vi "Dispense X Gallon at Y Flowrate.vi"(0 "Gallon Target":dbl=10.72, 1 "Equipment":T3={"COM Port"="COM1", "MW100"="MW100", "AG34970"="A-34972A", "Chamber"="WT500"}, 2 "Semiphore":T4, 5 "GPM Target":dbl=3.0, 11 "Error In":errorcluster, 12 "Test Condition":T1=enum."SRK500,Station1,5GPM FR", 13 "Ctl Refnum":refnum<vi>) -> (4 "M*-1":dbl, 6 "M*(Gallons)":dbl, 8 "ToutMax":dbl, 10 "ToutMin":dbl, 14 "POWER Ref":refnum<vi>, 15 "Error Out":errorcluster)   [LabVIEW 2009]
uses:
  PowerElements.ctl
  EquipReferences.ctl
  HEWH Tank Indicator.ctl
  TestedFlowratesScenarios.ctl
  Intellifaucet/Intellfaucet Mode.ctl
  ChannelSettings.ctl
panel:
  out "Tank Display":T2 {"TC6" format="%.2g"; "TIN" format="%.2g"; "TOUT" format="%.2g"; "Mean" format="%.2f"; "Std Dev" format="%.2f"; "TC5" format="%.2g"; "TC4" format="%.2g"; "TC3" format="%.2g"; "TC2" format="%.2g"; "TC1" format="%.2g"}
  out "String":string
  out "Flow":dbl=3.8899999999999997
  out "Flow Chart":dbl(graph)
  out "Local?":bool
  out "MW100":refnum<visa-resource-name>="MW100"
  out "POWER":T5
  out "Current Draw Start Time":dbl format="%.2f"
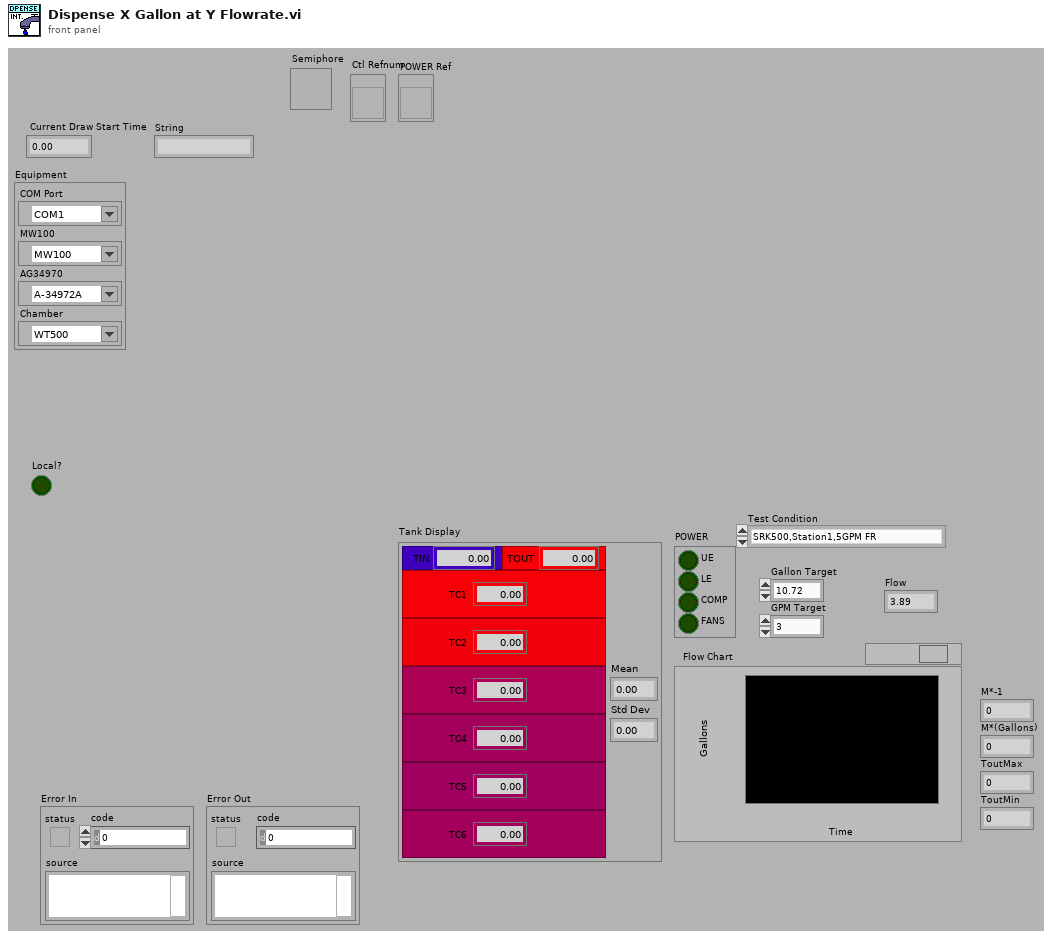
[diagram p1: front panel]
types:
  T1 = typedef "TestedFlowratesScenarios.ctl" = enum16{"DRK500,Station1", "DRK375,Lab", "SRK500,Station1,5GPM FR", "DRK375,STATION3,1/2\"HOSE", "DRK500,Station1,downspout", "DRK375,Station3,thruEcocute", "DRK375,Station3,purge", "Build2,2B,Purge", "Global, Purge", "Global, Tank"}
  T2 = typedef "HEWH Tank Indicator.ctl" = cluster{"TC1-D":bool, "TC2-D":bool, "TC3-D":bool, "TC4-D":bool, "TC5-D":bool, "RTD_IN":bool, "RTDOUT":bool, "TC1":dbl, "TC2":dbl, "TC3":dbl, "TC4":dbl, "TC5":dbl, "TIN":dbl, "TOUT":dbl, "Std Dev":dbl, "Mean":dbl, "TC6-D":bool, "TC6":dbl}
  T3 = typedef "EquipReferences.ctl" = cluster{"COM Port":refnum<visa-resource-name>, "MW100":refnum<visa-resource-name>, "AG34970":refnum<visa-resource-name>, "Chamber":refnum<visa-resource-name>}
  T4 = typedef "Semaphore RefNum" = refnum<k1>
  T5 = typedef "PowerElements.ctl" = cluster{"UE":bool, "LE":bool, "COMP":bool, "FANS":bool}
  T6 = typedef "Intellfaucet Mode.ctl" = enum16{"Adjust Temp", "Adjust Flow", "Start Flow", "Stop Flow"}
  T7 = typedef "ChannelSettings.ctl" = u32
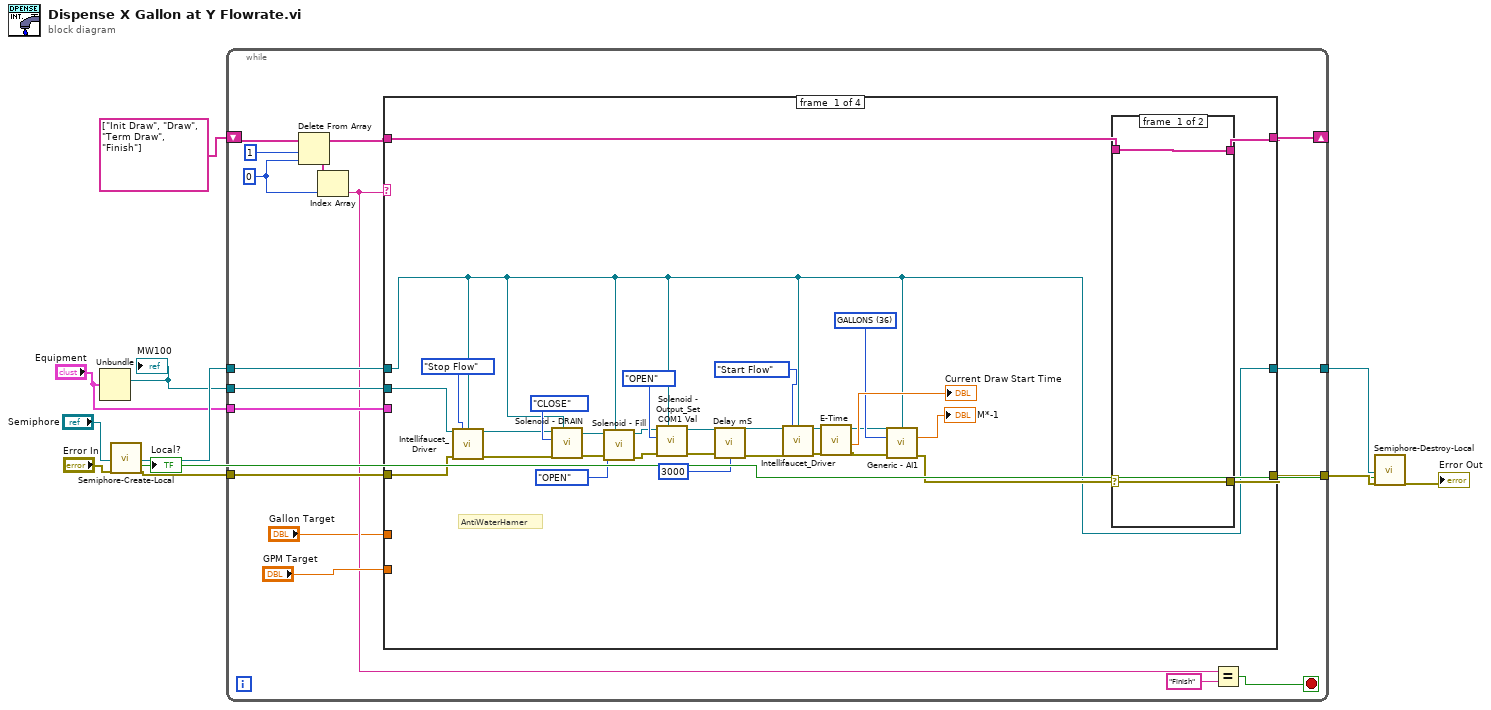
[diagram p0: block diagram]
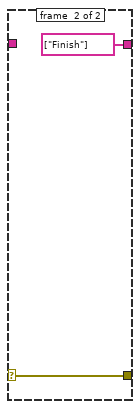
[diagram p2: hidden frame]
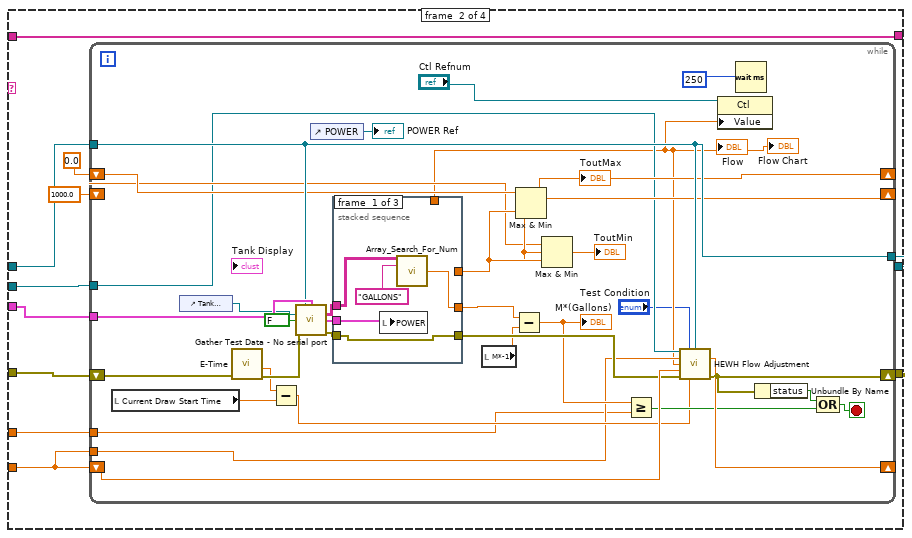
[diagram p3: hidden frame]
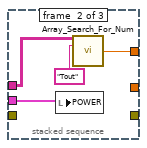
[diagram p4: hidden frame]
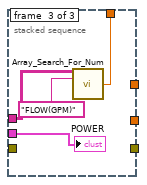
[diagram p5: hidden frame]
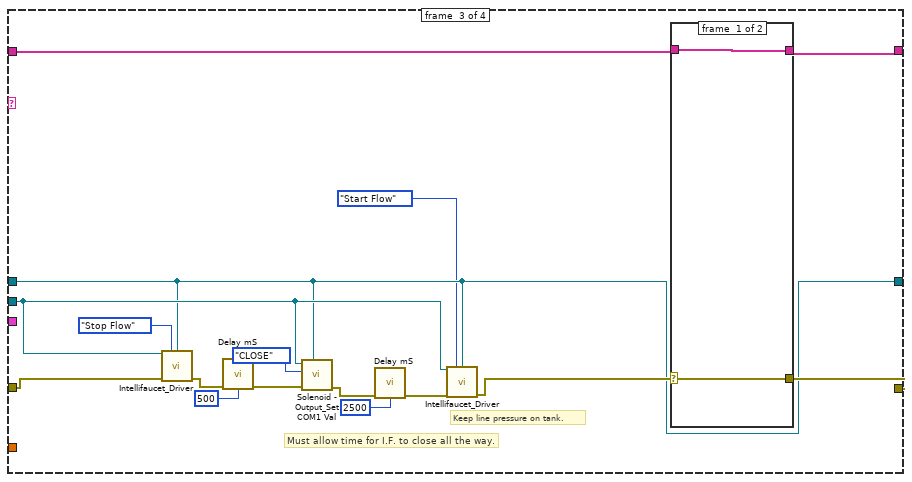
[diagram p6: hidden frame]
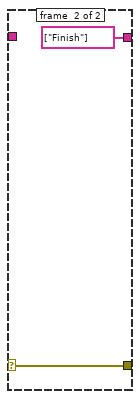
[diagram p7: hidden frame]
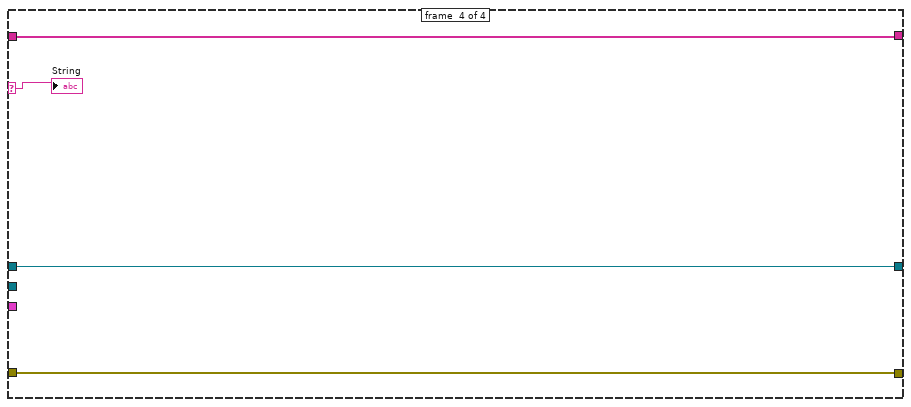
[diagram p8: hidden frame]
diagram:
  n1 = Unbundle("Equipment") -> ("MW100"=w5:refnum<visa-resource-name>)  [unwired: 3 out]
  "MW100" <- w5
  n2 = call "Semiphore-Create-Local.vi"("Semiphore"="Semiphore", "error in (no error)"="Error In") -> ("semaphore"=w8:T4, "Local?"=w1:bool, "error out"=w10:errorcluster)  [unwired: 15 in]
  "Local?" <- w1
  n3 = while {
    tunnel: w10 -> [w28]
    tunnel: w8 -> [w27]
    tunnel: "Equipment" -> [w21]
    tunnel: w5 -> [w20]
    tunnel: [w19] -> w4
    shift-right: [w17] -> _
    shift-left: string[] ["Init Draw", "Draw", "Term Draw", "Finish"] ("array") -> [w22]
    tunnel: [w12] -> w2
    stop <- w14 stop-if-true
    w24 = 0 ("index")
    n4 = Delete From Array(array=w22, length=1, index=w24) -> (deleted portion=w25:string[], array with subset deleted=w23:string[])
    n5 = Index Array(array=w25, index=w24) -> (element=w16:string)
    n6 = case shown="\"Term Draw\"" w16 {
      selector: w16 -> [_ _ _ w143]
      tunnel: [w55 w68 w133 w140] -> w17
      tunnel: w23 -> [w56 w68 w134 w140]
      tunnel: [w54 w70 w132 w141] -> w19
      tunnel: w28 -> [w38 w67 w131 w141]
      tunnel: w27 -> [w35 w71 w128 w142]
      tunnel: w21 -> [_ w65 _ _]
      tunnel: [w35 w66 w128 w142] -> w12
      tunnel: w20 -> [w37 w64 w129 _]
      tunnel: "GPM Target" -> [_ w62 _ _]
      tunnel: "Gallon Target" -> [_ w61 _ _]
      frame #0 {
        w48 = T7 36 items=["4-20_OUT", "Pres_HI1", "Pres_HI2", "Pres_LOW", "Pres_PIN", "HEATER_TOP", "HEATER_BOT", "T_Shell", "FLOWMETER", "WATT_SENSE", "WH_TICK", "Tc_1", "Tc_2", "Tc_3", "Tc_4", "Tc_5", "Tc_6", "Tc_down", "T_Shell_2", "T_Shell_3", "T_Shell_4", "RTD_IN", "RTD_OUT", "RTD_AMB", "INTF_TEMPFLO", "INTF_READY", "INTF_START", "INTF_STOP", "DRM_LOW", "DRM_HIGH", "PWR_MAIN", "VLV_DUMP", "VLV_OUT", "VLV_IN", "WATT_HOURS", "FLOW(SAMPLE)", "GALLONS", "FLOW(GPM)"] ("Channel_Enum")
        # "AntiWaterHamer"
        n7 = call "Intellifaucet_Driver.vi"("VISA session"=w37, "Mode"=Intellfaucet_Mode."Stop Flow", "Semiphore"=w35, "Error In"=w38) -> ("VISA session out"=w36:refnum<visa-resource-name>, "Error Out"=w32:errorcluster)  [unwired: 10 in]
        n8 = call "Solenoid - DRAIN.vi"("Semiphore"=w35, "Error In"=w32, "VALVE OPEN CLOSE"=enum8{"OPEN", "CLOSE"}."CLOSE", "VISA session"=w36) -> ("Error Out"=w43:errorcluster, "dup VISA session"=w40:refnum<visa-resource-name>)  [unwired: 6 in]
        n9 = call "Solenoid - Fill.vi"("Semiphore"=w35, "Error In"=w43, "VALVE OPEN CLOSE"=enum8{"OPEN", "CLOSE"}."OPEN", "VISA session"=w40) -> ("Error Out"=w42:errorcluster, "dup VISA session"=w41:refnum<visa-resource-name>)  [unwired: 6 in]
        n10 = call "Solenoid - Output_Set COM1 Val.vi"("Semiphore"=w35, "Error In"=w42, "OPEN CLOSE"=enum8{"CLOSE", "OPEN"}."OPEN", "VISA session"=w41) -> ("Error Out"=w31:errorcluster, "dup VISA session"=w49:refnum<visa-resource-name>)  [unwired: 6 in]
        n11 = call "Delay mS.vi"("Error In"=w31, "milliseconds to wait"=u32 3000) -> ("Error Out"=w30:errorcluster)  [unwired: 13 in]
        n12 = call "Intellifaucet_Driver.vi"("VISA session"=w49, "Mode"=Intellfaucet_Mode."Start Flow", "Semiphore"=w35, "Error In"=w30) -> ("VISA session out"=w46:refnum<visa-resource-name>, "Error Out"=w50:errorcluster)  [unwired: 10 in]
        n13 = call "E-Time.vi"("error in (no error)"=w50) -> ("error out"=w44:errorcluster, "Elapsed Time (sec)"=→"Current Draw Start Time":dbl)  [unwired: 8 in, 1 out]
        n14 = call "Generic - AI1.vi"("MW100"=w46, "Semiphore"=w35, "Channel_Enum"=w48, "Error In"=w44) -> ("Value"=→"M*-1":dbl, "Error Out"=w45:errorcluster)  [unwired: 9 in, 1 out]
        n15 = case shown="No Error" w45 {
          selector: w45 -> [w57 w60]
          tunnel: [w58 string[] ["Finish"] ("States")] -> w55
          tunnel: w56 -> [w58 _]
          tunnel: [w57 w60] -> w54
          frame #0 {
          }
          frame #1 {
          }
        }
      }
      frame #1 {
        n16 = while {
          shift-right: [w95] -> w70
          shift-left: w67 -> [w78]
          shift-right: [w104] -> _
          shift-left: w62 -> [w105]
          tunnel: w71 -> [w96]
          tunnel: [w96] -> w66
          shift-right: [w86] -> _
          shift-left: 0.0 ("GPM") -> [w87]
          tunnel: w65 -> [w99]
          tunnel: w64 -> [w82]
          shift-right: [w84] -> _
          shift-left: 1000.0 -> [w83]
          tunnel: w62 -> [w79]
          tunnel: w61 -> [w77]
          stop <- w106 stop-if-true
          n17 = local read "Current Draw Start Time"() -> (w81:dbl)
          n18 = control-ref of="Tank Display"() -> (w73:refnum<vi>)
          n19 = call "E-Time.vi"("error in (no error)"=w78) -> ("error out"=w102:errorcluster, "Elapsed Time (sec)"=w98:dbl)  [unwired: 8 in, 1 out]
          n20 = Subtract(x=w98, y=w81) -> (x-y=w97:dbl)
          n21 = call "Gather Test Data - No serial port.vi"("Semiphore"=w96, "Equipment"=w99, "Tank Display Ref"=w73, "Agilent?"=FALSE, "error in (no error)"=w102) -> ("Output Data"=w92:string[][], "POWER"=w89:T5, "error out"=w93:errorcluster)  [unwired: 6 in, 2 out]
          n22 = control-ref of="POWER"() -> (→"POWER Ref":refnum<vi>)
          n23 = stacked-sequence {
            tunnel: w93 -> [w107 _ _]
            tunnel: w92 -> [w110 w114 w119]
            tunnel: [w108 _ _] -> w90
            tunnel: [w107 _ _] -> w101
            tunnel: w89 -> [w111 w115 w116]
            tunnel: [_ w112 _] -> w85
            tunnel: [_ _ w117] -> w74
            frame #0 {
              n24 = local write "POWER"(w111) -> ()
              n25 = call "Array_Search_For_Num.vi"("N Rows of Data"=w110, "Title?"="GALLONS") -> ("number"=w108:dbl)  [unwired: 12 in, 1 out]
            }
            frame #1 {
              n26 = local write "POWER"(w115) -> ()
              n27 = call "Array_Search_For_Num.vi"("N Rows of Data"=w114, "Title?"="Tout") -> ("number"=w112:dbl)  [unwired: 12 in, 1 out]
            }
            frame #2 {
              n28 = call "Array_Search_For_Num.vi"("N Rows of Data"=w119, "Title?"="FLOW(GPM)") -> ("number"=w117:dbl)  [unwired: 12 in, 1 out]
              "POWER" <- w116
            }
          }
          "Flow" <- w74
          "Flow Chart" <- w74
          n29 = local read "M*-1"() -> (w91:dbl)
          n30 = Subtract(x=w90, y=w91) -> (x-y=w80:dbl)
          "M*(Gallons)" <- w80
          n31 = Max & Min(x=w87, y=w85) -> (max(x,y)=w86:dbl)  [unwired: 1 out]
          "ToutMax" <- w86
          n32 = Max & Min(x=w83, y=w85) -> (min(x,y)=w84:dbl)  [unwired: 1 out]
          "ToutMin" <- w84
          n33 = Greater Or Equal?(x=w80, y=w77) -> (x >= y?=w100:bool)
          n34 = call "HEWH Flow Adjustment.vi"("VISA session"=w82, "Configuration"="Test Condition", "Semiphore"=w96, "GPM Target(3)"=w79, "GPM reading"=w74, "Flow rate setting In"=w105, "Error In"=w101, "Elapsed Time (sec)"=w97) -> ("Flow rate setting Out"=w104:dbl, "Error Out"=w95:errorcluster)  [unwired: 5 in, 1 out]
          n35 = property class="Ctl"(reference="Ctl Refnum", "Value"=w74) -> ()  [unwired: 1 in, 2 out]
          n36 = Wait (ms)(milliseconds to wait=u32 250) -> ()  [unwired: 1 out]
          n37 = Unbundle By Name(w95) -> ("status"=w103:bool)
          n38 = Compound Arithmetic op=OR(w103, w100) -> (w106:bool)
        }
      }
      frame #2 {
        # "Must allow time for I.F. to close all the way."
        # "Keep line pressure on tank."
        n39 = call "Intellifaucet_Driver.vi"("VISA session"=w129, "Mode"=Intellfaucet_Mode."Stop Flow", "Semiphore"=w128, "Error In"=w131) -> ("Error Out"=w126:errorcluster)  [unwired: 10 in, 1 out]
        n40 = call "Delay mS.vi"("Error In"=w126, "milliseconds to wait"=u32 500) -> ("Error Out"=w125:errorcluster)  [unwired: 13 in]
        n41 = call "Solenoid - Output_Set COM1 Val.vi"("Semiphore"=w128, "Error In"=w125, "OPEN CLOSE"=enum8{"CLOSE", "OPEN"}."CLOSE", "VISA session"=w129) -> ("Error Out"=w121:errorcluster)  [unwired: 6 in, 1 out]
        n42 = call "Delay mS.vi"("Error In"=w121, "milliseconds to wait"=u32 2500) -> ("Error Out"=w120:errorcluster)  [unwired: 13 in]
        n43 = call "Intellifaucet_Driver.vi"("VISA session"=w129, "Mode"=Intellfaucet_Mode."Start Flow", "Semiphore"=w128, "Error In"=w120) -> ("Error Out"=w130:errorcluster)  [unwired: 10 in, 1 out]
        n44 = case shown="Error" w130 {
          selector: w130 -> [w136 w139]
          tunnel: [w137 string[] ["Finish"] ("States")] -> w133
          tunnel: w134 -> [w137 _]
          tunnel: [w136 w139] -> w132
          frame #0 {
          }
          frame #1 {
          }
        }
      }
      frame #3 {
        "String" <- w143
      }
    }
    n45 = Equal?(x=w16, y="Finish") -> (x = y?=w14:bool)
  }
  n46 = call "Semiphore-Destroy-Local.vi"("Semiphore"=w2, "Local?"=w1, "error in (no error)"=w4) -> ("error out"=→"Error Out":errorcluster)  [unwired: 16 in]
